vi "control.vi"() -> ()   [LabVIEW 2020]
uses:
  Pos_modifi.vi
  Llenado.vi
  sensores.vi
panel:
  in  "stop":bool
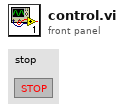
[diagram p1: front panel]
types:
  T1 = cluster{"Sensor 1":bool, "Laminadora":bool, "PistonA":bool, "PistonC":bool}
  T2 = cluster{"Pos_Car":dbl, "Pos_lataAb":dbl, "Pos_lataCd":dbl, "Pos_lataPtd":dbl}
  T3 = cluster{"Bote":u8, "Llenador":u8, "Tanque":u8, "Pintado":dbl, "Mezclador":dbl}
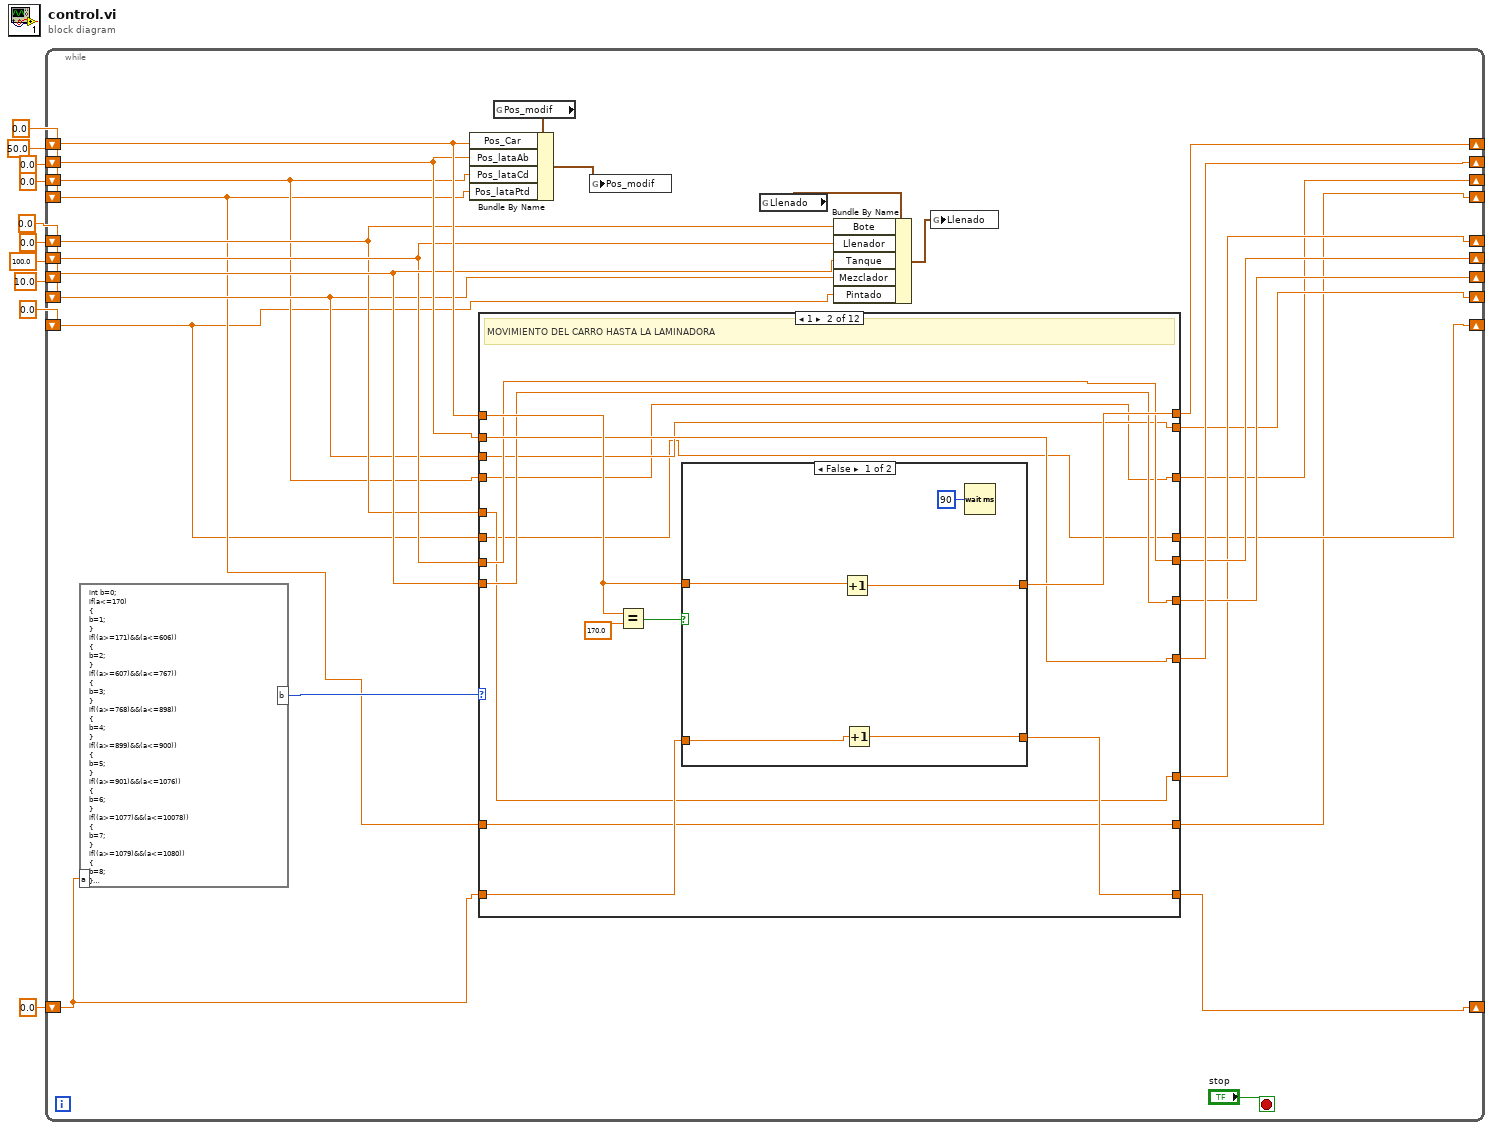
[diagram p0: block diagram]
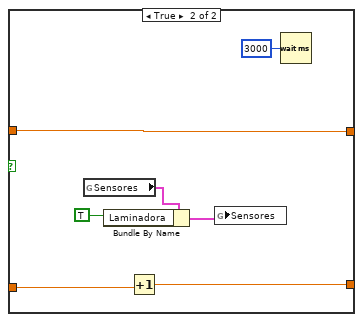
[diagram p3: hidden frame]
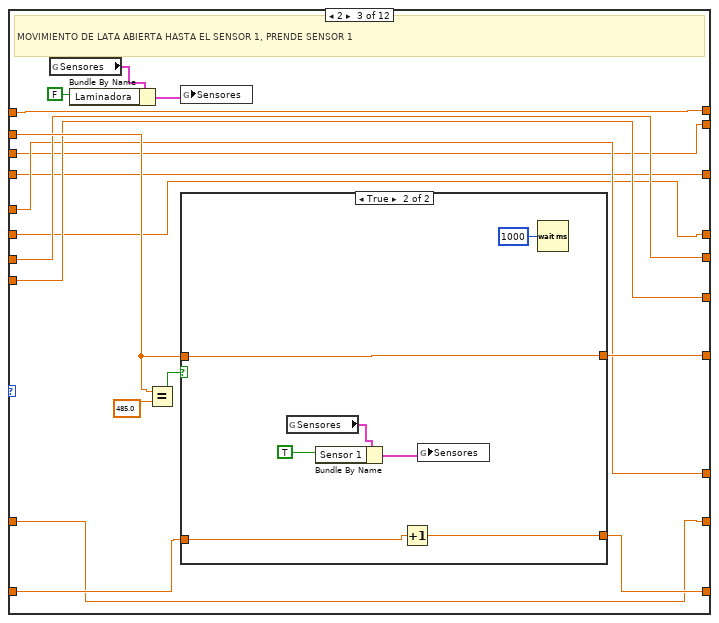
[diagram p4: hidden frame]
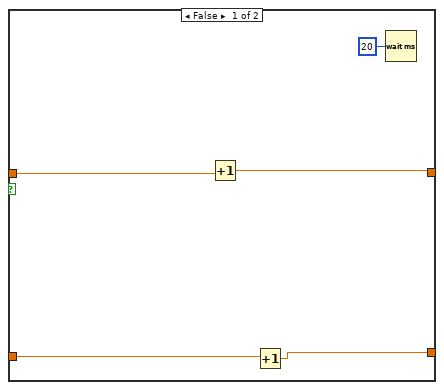
[diagram p5: hidden frame]
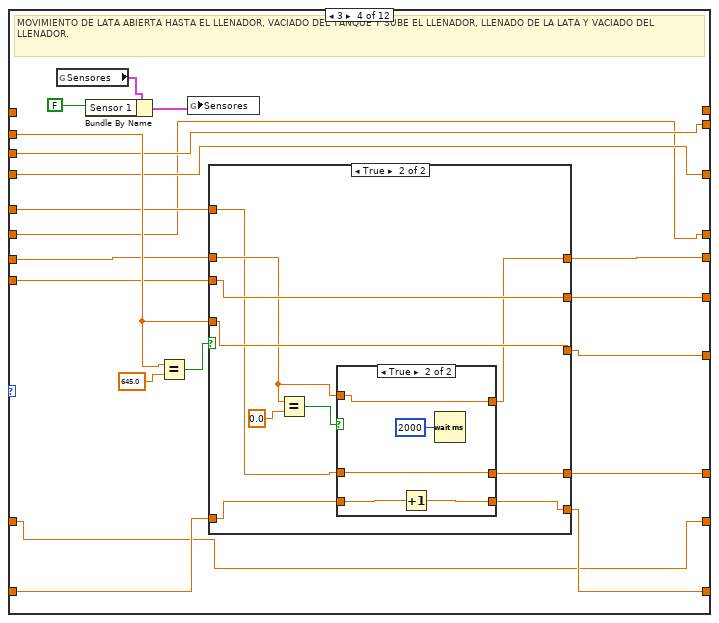
[diagram p6: hidden frame]
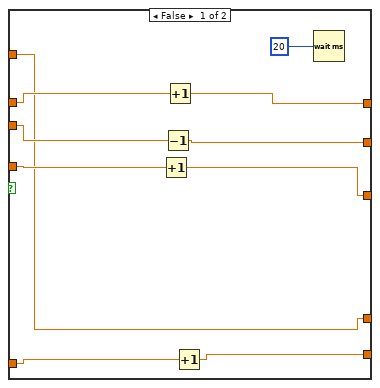
[diagram p7: hidden frame]
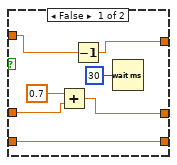
[diagram p8: hidden frame]
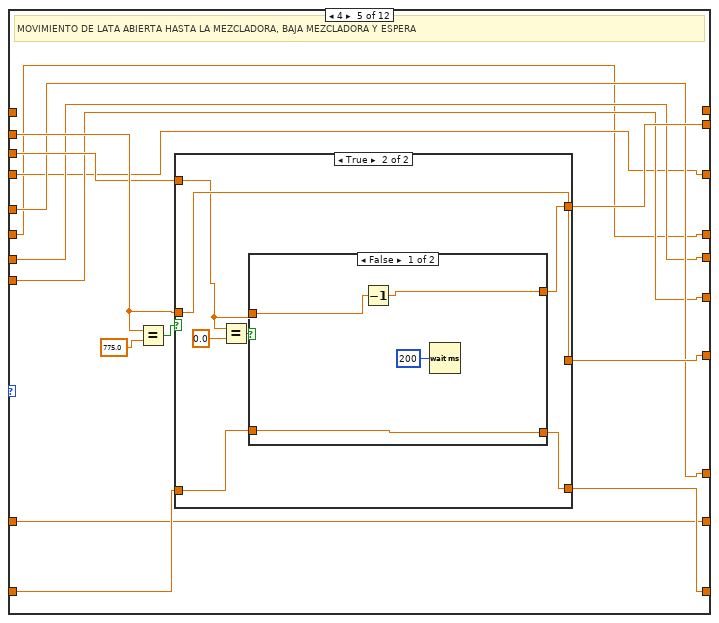
[diagram p9: hidden frame]
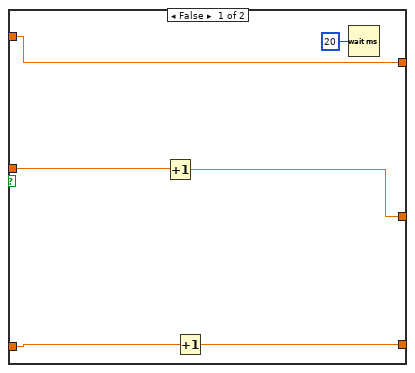
[diagram p10: hidden frame]
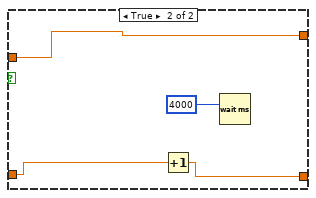
[diagram p11: hidden frame]
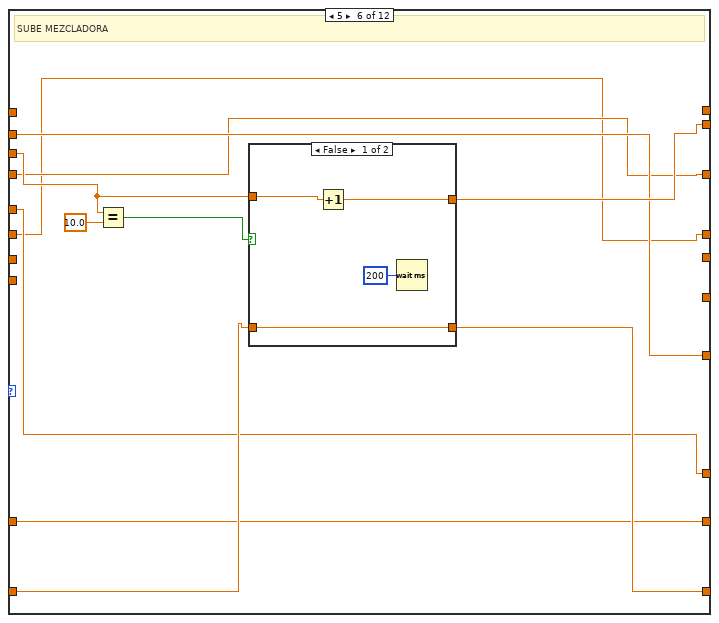
[diagram p12: hidden frame]
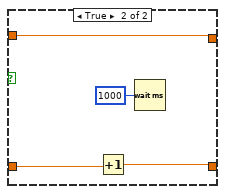
[diagram p13: hidden frame]
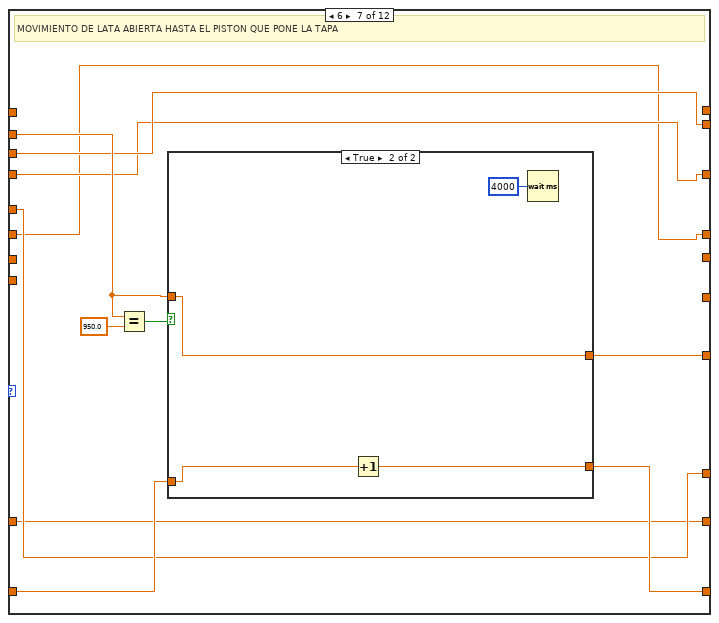
[diagram p14: hidden frame]
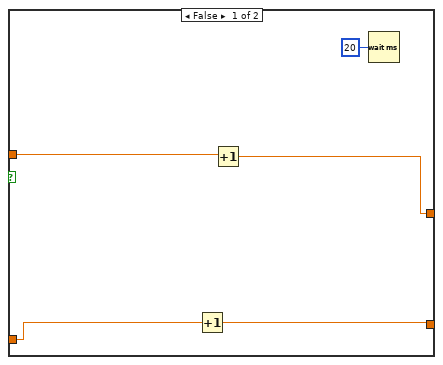
[diagram p15: hidden frame]
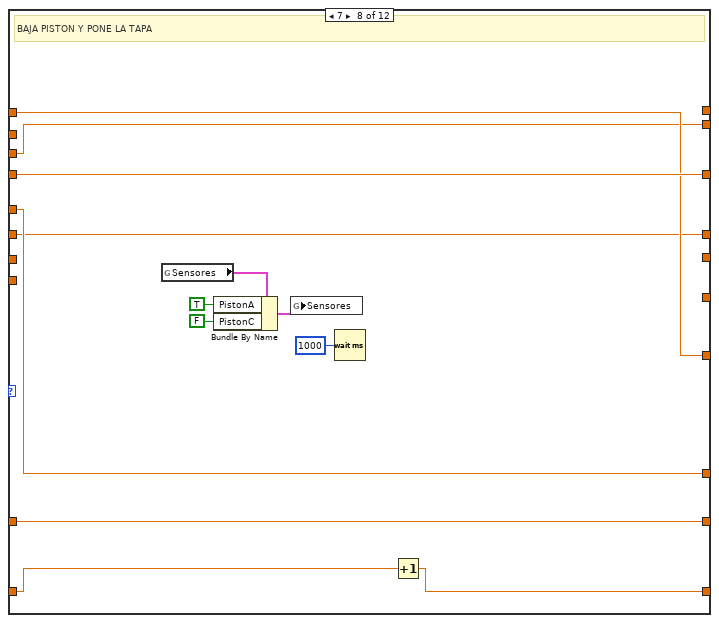
[diagram p16: hidden frame]
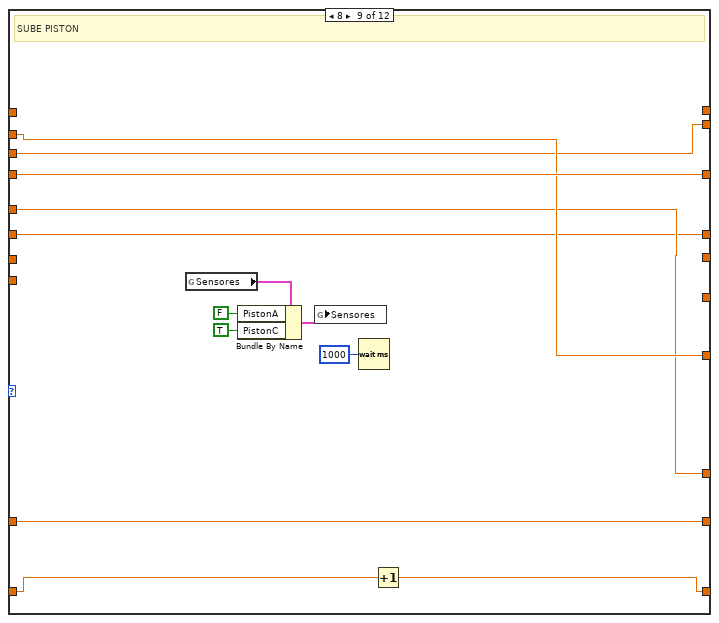
[diagram p17: hidden frame]
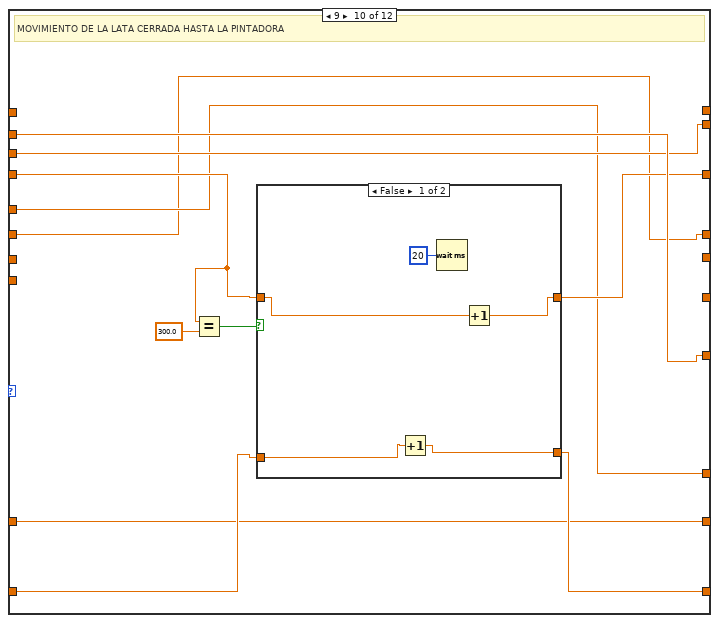
[diagram p18: hidden frame]
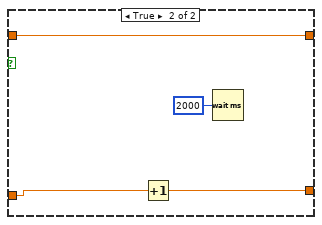
[diagram p19: hidden frame]
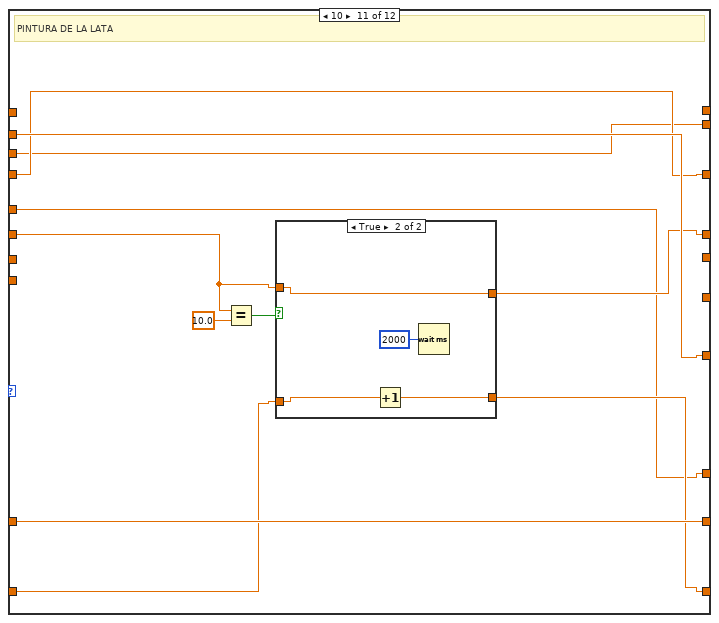
[diagram p20: hidden frame]
diagram:
  n1 = while {
    shift-right: [w29] -> _
    shift-left: 0.0 -> [w30]
    shift-right: [w31] -> _
    shift-left: 0.0 -> [w32]
    shift-right: [w27] -> _
    shift-left: 50.0 -> [w28]
    shift-right: [w21] -> _
    shift-left: 0.0 -> [w23]
    shift-right: [w22] -> _
    shift-left: 100.0 -> [w24]
    shift-right: [w19] -> _
    shift-left: 0.0 -> [w20]
    shift-right: [w17] -> _
    shift-left: 10.0 -> [w18]
    shift-right: [w15] -> _
    shift-left: 0.0 -> [w16]
    shift-right: [w11] -> _
    shift-left: 0.0 -> [w14]
    shift-right: [w12] -> _
    shift-left: 0.0 -> [w13]
    stop <- "stop" stop-if-true
    n2 = formula code="int b=0;\nif(a<=170)\n{\nb=1;\n}\nif((a>=171)&&(a<=606))\n{\nb=2;\n}\nif((a>=607)&&(a<=767))\n{\nb=3;\n}\nif((a>=768)&&(a<=898))\n{\nb=4;\n}\nif((a>=899)&&(a<=900))\n{\nb=5;\n}\nif((a>=901)&&(a<=1076))\n{\nb=6;\n}\nif((a>=1077)&&(a<=10078))\n{\nb=7;\n}\nif((a>=1079)&&(a<=1080))\n{\nb=8;\n}\nif((a>=1081)&&(a<=1381))\n{\nb=9;\n}\nif((a>=1382)&&(a<=1392))\n{\nb=10;\n}\nif((a>=1393)&&(a<=13292))\n{\nb=11;\n}"("a"=w30) -> ("b"=w35:i32)
    n3 = case shown="1" w35 {
      tunnel: w32 -> [w46 w58 w85 _ _ _ _ w238 _ _ _ _]
      tunnel: [w46 w57 w85 _ _ _ _ _ _ _ _ _] -> w31
      tunnel: w30 -> [w45 w56 w84 w113 w164 w195 w214 w237 w246 w257 w276 w300]
      tunnel: [w45 w55 w83 w112 w163 w194 w213 w236 w245 w256 w275 w299] -> w29
      tunnel: w28 -> [w44 w54 w82 w115 w162 w192 w215 _ w244 w263 w282 w297]
      tunnel: [w44 w54 w81 w114 w161 w192 w212 w238 w244 w263 w282 w297] -> w27
      tunnel: w24 -> [w42 w52 w78 w111 w156 _ _ _ _ _ _ _]
      tunnel: w23 -> [w43 w53 w79 w110 w157 _ _ _ _ _ _ _]
      tunnel: [w43 w53 w79 w109 w157 _ _ _ _ _ _ _] -> w21
      tunnel: [w42 w52 w78 w108 w156 _ _ _ _ _ _ _] -> w22
      tunnel: w20 -> [w41 w51 w77 w107 w158 w190 w209 w229 w242 w255 w273 w293]
      tunnel: [w41 w51 w77 w106 w158 w190 w209 w229 w242 w255 w273 w293] -> w19
      tunnel: w18 -> [w40 w50 w76 w105 w160 w196 w211 w235 w243 w262 w274 w296]
      tunnel: [w40 w50 w76 w105 w159 w193 w211 w235 w243 w262 w274 w296] -> w17
      tunnel: w16 -> [w39 w49 w75 w104 w155 w191 w210 w239 w247 w259 w281 w295]
      tunnel: [w39 w49 w75 w104 w155 w191 w210 w239 w247 w258 w281 w295] -> w15
      tunnel: w14 -> [w37 w47 w73 w102 w153 w188 w207 w227 w240 w253 w283 w301]
      tunnel: w13 -> [w38 w48 w74 w103 w154 w189 w208 w228 w241 w254 w278 w294]
      tunnel: [w38 w48 w74 w103 w154 w189 w208 w228 w241 w254 w277 w294] -> w12
      tunnel: [w37 w47 w73 w102 w153 w188 w207 w227 w240 w253 w283 w298] -> w11
      frame 0, Default {
      }
      frame 1 {
        # "MOVIMIENTO DEL CARRO HASTA LA LAMINADORA"
        n4 = Equal?(x=w58, y=170.0) -> (x = y?=w60:bool)
        n5 = case shown="False" w60 {
          tunnel: w58 -> [w62 w69]
          tunnel: [w61 w69] -> w57
          tunnel: w56 -> [w65 w72]
          tunnel: [w64 w71] -> w55
          frame False {
            n6 = Increment(x=w62) -> (x+1=w61:dbl)
            n7 = Increment(x=w65) -> (x+1=w64:dbl)
            n8 = Wait (ms)(milliseconds to wait=u32 90) -> ()  [unwired: 1 out]
          }
          frame True {
            n9 = global read "sensores.vi" "Sensores"() -> (w68:T1)
            n10 = Bundle By Name(cluster=w68, "Laminadora"=TRUE ("Sensor 1")) -> (w67:T1)
            n11 = Increment(x=w72) -> (x+1=w71:dbl)
            n12 = global write "sensores.vi" "Sensores"(w67) -> ()
            n13 = Wait (ms)(milliseconds to wait=u32 3000) -> ()  [unwired: 1 out]
          }
        }
      }
      frame 2 {
        # "MOVIMIENTO DE LATA ABIERTA HASTA EL SENSOR 1, PRENDE SENSOR 1"
        n14 = global read "sensores.vi" "Sensores"() -> (w88:T1)
        n15 = Bundle By Name(cluster=w88, "Laminadora"=FALSE ("Sensor 1")) -> (w89:T1)
        n16 = Equal?(x=w82, y=485.0) -> (x = y?=w80:bool)
        n17 = global write "sensores.vi" "Sensores"(w89) -> ()
        n18 = case shown="True" w80 {
          tunnel: w84 -> [w94 w101]
          tunnel: [w93 w100] -> w83
          tunnel: w82 -> [w92 w99]
          tunnel: [w91 w99] -> w81
          frame False {
            n19 = Increment(x=w92) -> (x+1=w91:dbl)
            n20 = Increment(x=w94) -> (x+1=w93:dbl)
            n21 = Wait (ms)(milliseconds to wait=u32 20) -> ()  [unwired: 1 out]
          }
          frame True {
            n22 = global read "sensores.vi" "Sensores"() -> (w97:T1)
            n23 = Bundle By Name(cluster=w97, "Sensor 1"=TRUE) -> (w96:T1)
            n24 = Increment(x=w101) -> (x+1=w100:dbl)
            n25 = global write "sensores.vi" "Sensores"(w96) -> ()
            n26 = Wait (ms)(milliseconds to wait=u32 1000) -> ()  [unwired: 1 out]
          }
        }
      }
      frame 3 {
        # "MOVIMIENTO DE LATA ABIERTA HASTA EL LLENADOR, VACIADO DEL TANQUE Y SUBE EL LLENADOR, LLENADO DE LA LATA Y VACIADO DEL LLENADOR."
        n27 = global read "sensores.vi" "Sensores"() -> (w118:T1)
        n28 = Bundle By Name(cluster=w118, "Sensor 1"=FALSE) -> (w119:T1)
        n29 = Equal?(x=w115, y=645.0) -> (x = y?=w116:bool)
        n30 = global write "sensores.vi" "Sensores"(w119) -> ()
        n31 = case shown="True" w116 {
          tunnel: w115 -> [w130 w140]
          tunnel: [w129 w140] -> w114
          tunnel: w113 -> [w128 w137]
          tunnel: [w127 w136] -> w112
          tunnel: w111 -> [w123 w139]
          tunnel: w110 -> [w125 w134]
          tunnel: [w124 w133] -> w109
          tunnel: [w122 w139] -> w108
          tunnel: w107 -> [w121 w132]
          tunnel: [w121 w131] -> w106
          frame False {
            n32 = Increment(x=w130) -> (x+1=w129:dbl)
            n33 = Decrement(x=w123) -> (x-1=w122:dbl)
            n34 = Increment(x=w125) -> (x+1=w124:dbl)
            n35 = Increment(x=w128) -> (x+1=w127:dbl)
            n36 = Wait (ms)(milliseconds to wait=u32 20) -> ()  [unwired: 1 out]
          }
          frame True {
            n37 = Equal?(x=w134, y=0.0) -> (x = y?=w135:bool)
            n38 = case shown="True" w135 {
              tunnel: w137 -> [w147 w152]
              tunnel: [w147 w151] -> w136
              tunnel: w134 -> [w146 w150]
              tunnel: [w145 w150] -> w133
              tunnel: w132 -> [w141 w148]
              tunnel: [w143 w148] -> w131
              frame False {
                n39 = Add(x=0.7, y=w141) -> (x+y=w143:dbl)
                n40 = Decrement(x=w146) -> (x-1=w145:dbl)
                n41 = Wait (ms)(milliseconds to wait=u32 30) -> ()  [unwired: 1 out]
              }
              frame True {
                n42 = Increment(x=w152) -> (x+1=w151:dbl)
                n43 = Wait (ms)(milliseconds to wait=u32 2000) -> ()  [unwired: 1 out]
              }
            }
          }
        }
      }
      frame 4 {
        # "MOVIMIENTO DE LATA ABIERTA HASTA LA MEZCLADORA, BAJA MEZCLADORA Y ESPERA"
        n44 = Equal?(x=w162, y=775.0) -> (x = y?=w165:bool)
        n45 = case shown="True" w165 {
          tunnel: w164 -> [w172 w176]
          tunnel: [w171 w175] -> w163
          tunnel: w162 -> [w170 w179]
          tunnel: [w169 w179] -> w161
          tunnel: w160 -> [w167 w173]
          tunnel: [w167 w174] -> w159
          frame False {
            n46 = Increment(x=w170) -> (x+1=w169:dbl)
            n47 = Increment(x=w172) -> (x+1=w171:dbl)
            n48 = Wait (ms)(milliseconds to wait=u32 20) -> ()  [unwired: 1 out]
          }
          frame True {
            n49 = Equal?(x=w173, y=0.0) -> (x = y?=w177:bool)
            n50 = case shown="False" w177 {
              tunnel: w173 -> [w181 w184]
              tunnel: w176 -> [w183 w186]
              tunnel: [w183 w185] -> w175
              tunnel: [w182 w184] -> w174
              frame False {
                n51 = Decrement(x=w181) -> (x-1=w182:dbl)
                n52 = Wait (ms)(milliseconds to wait=u32 200) -> ()  [unwired: 1 out]
              }
              frame True {
                n53 = Increment(x=w186) -> (x+1=w185:dbl)
                n54 = Wait (ms)(milliseconds to wait=u32 4000) -> ()  [unwired: 1 out]
              }
            }
          }
        }
      }
      frame 5 {
        # "SUBE MEZCLADORA"
        n55 = Equal?(x=w196, y=10.0) -> (x = y?=w197:bool)
        n56 = case shown="False" w197 {
          tunnel: w196 -> [w202 w206]
          tunnel: [w201 w206] -> w193
          tunnel: w195 -> [w199 w205]
          tunnel: [w199 w204] -> w194
          frame False {
            n57 = Increment(x=w202) -> (x+1=w201:dbl)
            n58 = Wait (ms)(milliseconds to wait=u32 200) -> ()  [unwired: 1 out]
          }
          frame True {
            n59 = Increment(x=w205) -> (x+1=w204:dbl)
            n60 = Wait (ms)(milliseconds to wait=u32 1000) -> ()  [unwired: 1 out]
          }
        }
      }
      frame 6 {
        # "MOVIMIENTO DE LATA ABIERTA HASTA EL PISTON QUE PONE LA TAPA"
        n61 = Equal?(x=w215, y=950.0) -> (x = y?=w217:bool)
        n62 = case shown="True" w217 {
          tunnel: w215 -> [w222 w224]
          tunnel: w214 -> [w220 w226]
          tunnel: [w219 w225] -> w213
          tunnel: [w221 w224] -> w212
          frame False {
            n63 = Increment(x=w220) -> (x+1=w219:dbl)
            n64 = Increment(x=w222) -> (x+1=w221:dbl)
            n65 = Wait (ms)(milliseconds to wait=u32 20) -> ()  [unwired: 1 out]
          }
          frame True {
            n66 = Increment(x=w226) -> (x+1=w225:dbl)
            n67 = Wait (ms)(milliseconds to wait=u32 4000) -> ()  [unwired: 1 out]
          }
        }
      }
      frame 7 {
        # "BAJA PISTON Y PONE LA TAPA"
        n68 = global read "sensores.vi" "Sensores"() -> (w234:T1)
        n69 = Bundle By Name(cluster=w234, "PistonA"=TRUE, "PistonC"=FALSE) -> (w233:T1)
        n70 = global write "sensores.vi" "Sensores"(w233) -> ()
        n71 = Wait (ms)(milliseconds to wait=u32 1000) -> ()  [unwired: 1 out]
        n72 = Increment(x=w237) -> (x+1=w236:dbl)
      }
      frame 8 {
        # "SUBE PISTON"
        n73 = global read "sensores.vi" "Sensores"() -> (w252:T1)
        n74 = Bundle By Name(cluster=w252, "PistonA"=FALSE, "PistonC"=TRUE) -> (w251:T1)
        n75 = global write "sensores.vi" "Sensores"(w251) -> ()
        n76 = Wait (ms)(milliseconds to wait=u32 1000) -> ()  [unwired: 1 out]
        n77 = Increment(x=w246) -> (x+1=w245:dbl)
      }
      frame 9 {
        # "MOVIMIENTO DE LA LATA CERRADA HASTA LA PINTADORA"
        n78 = Equal?(x=w259, y=300.0) -> (x = y?=w261:bool)
        n79 = case shown="False" w261 {
          tunnel: w259 -> [w267 w272]
          tunnel: [w268 w272] -> w258
          tunnel: w257 -> [w265 w271]
          tunnel: [w264 w270] -> w256
          frame False {
            n80 = Increment(x=w265) -> (x+1=w264:dbl)
            n81 = Wait (ms)(milliseconds to wait=u32 20) -> ()  [unwired: 1 out]
            n82 = Increment(x=w267) -> (x+1=w268:dbl)
          }
          frame True {
            n83 = Increment(x=w271) -> (x+1=w270:dbl)
            n84 = Wait (ms)(milliseconds to wait=u32 2000) -> ()  [unwired: 1 out]
          }
        }
      }
      frame 10 {
        # "PINTURA DE LA LATA"
        n85 = Equal?(x=w278, y=10.0) -> (x = y?=w280:bool)
        n86 = case shown="True" w280 {
          tunnel: w278 -> [w285 w292]
          tunnel: [w286 w292] -> w277
          tunnel: w276 -> [w287 w291]
          tunnel: [w288 w290] -> w275
          frame False {
            n87 = Increment(x=w287) -> (x+1=w288:dbl)
            n88 = Increment(x=w285) -> (x+1=w286:dbl)
            n89 = Wait (ms)(milliseconds to wait=u32 200) -> ()  [unwired: 1 out]
          }
          frame True {
            n90 = Increment(x=w291) -> (x+1=w290:dbl)
            n91 = Wait (ms)(milliseconds to wait=u32 2000) -> ()  [unwired: 1 out]
          }
        }
      }
      frame 11 {
        # "MOVIMIENTO DE LA LATA PINTADA HASTA LA CAJA"
        n92 = Equal?(x=w301, y=300.0) -> (x = y?=w303:bool)
        n93 = case shown="False" w303 {
          tunnel: w301 -> [w305 w310]
          tunnel: w300 -> [w308 w312]
          tunnel: [w307 w311] -> w299
          tunnel: [w306 w310] -> w298
          frame False {
            n94 = Increment(x=w308) -> (x+1=w307:dbl)
            n95 = Increment(x=w305) -> (x+1=w306:dbl)
            n96 = Wait (ms)(milliseconds to wait=u32 20) -> ()  [unwired: 1 out]
          }
          frame True {
            n97 = Increment(x=w312) -> (x+1=w311:dbl)
            n98 = Wait (ms)(milliseconds to wait=u32 4000) -> ()  [unwired: 1 out]
          }
        }
      }
    }
    n99 = global read "Pos_modifi.vi" "Pos_modif"() -> (w34:T2)
    n100 = Bundle By Name(cluster=w34, "Pos_Car"=w32, "Pos_lataAb"=w28, "Pos_lataCd"=w16, "Pos_lataPtd"=w14) -> (w33:T2)
    n101 = global write "Pos_modifi.vi" "Pos_modif"(w33) -> ()
    n102 = global read "Llenado.vi" "Llenado"() -> (w26:T3)
    n103 = Bundle By Name(cluster=w26, "Bote"=w20, "Llenador"=w23, "Tanque"=w24, "Mezclador"=w18, "Pintado"=w13) -> (w25:T3)
    n104 = global write "Llenado.vi" "Llenado"(w25) -> ()
  }
